vi "sequencedStringArray.vi"(8 "error in (no error)":errorcluster, 11 "ScriptEventList in":refnum<class "ScriptEventList.lvclass">) -> (0 "error out":errorcluster, 2 "eventStringArray":string[][](array[string]), 3 "ScriptEventList out":refnum<class "ScriptEventList.lvclass">)   [LabVIEW 2009, in "Tools.lvlib" / "Scripting.lvlib" / "ScriptEventList.lvclass"]
uses:
  ScriptEventList.lvclass
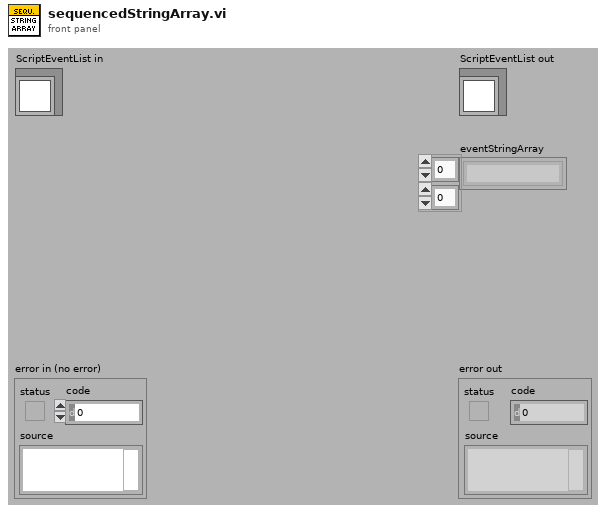
[diagram p1: front panel]
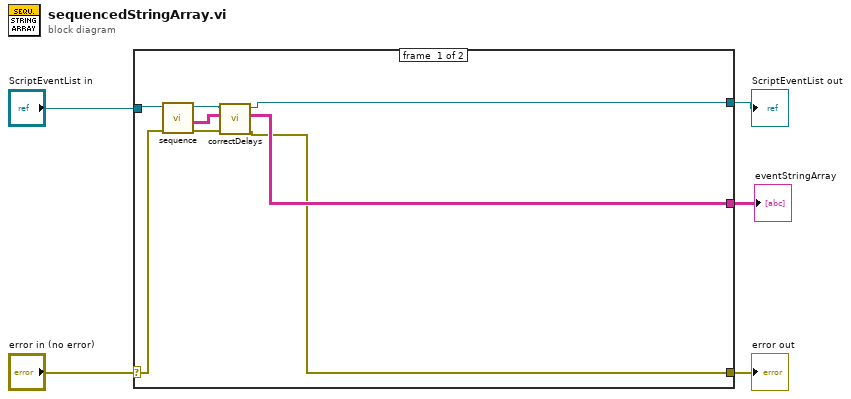
[diagram p0: block diagram]
diagram:
  n1 = case shown="No Error" "error in (no error)" {
    selector: "error in (no error)" -> [w12 w15]
    tunnel: [w6 w15] -> w4
    tunnel: [w7 w14] -> w2
    tunnel: "ScriptEventList in" -> [w13 w14]
    tunnel: [w8 _] -> w1
    frame #0 {
      n2 = call "sequence.vi"("error in (no error)"=w12, "ScriptEventList in"=w13) -> ("error out"=w11:errorcluster, "allStrings"=w9:string[][], "ScriptEventList out"=w10:refnum<class "ScriptEventList.lvclass">)  [unwired: 6 in, 1 out]
      n3 = call "correctDelays.vi"("error in (no error)"=w11, "eventStringArray in"=w9, "ScriptEventList in"=w10) -> ("error out"=w6:errorcluster, "eventStringArray"=w8:string[][], "ScriptEventList out"=w7:refnum<class "ScriptEventList.lvclass">)  [unwired: 6 in]
    }
    frame #1 {
    }
  }
  "error out" <- w4
  "ScriptEventList out" <- w2
  "eventStringArray" <- w1
